vi "FPGAsimpleTDC.vi"() -> ()   [LabVIEW 2017]
uses:
  <vilib>/Platform/TimedLoop/XDataNode/timing_clust.ctl
  <vilib>/Platform/TimedLoop/XDataNode/nitl_modes.ctl
  <vilib>/Platform/TimedLoop/XDataNode/wakeup.ctl
  <vilib>/rvi/Emulation/niFpgaGetClockAttributes.vi
  <vilib>/rvi/Emulation/niFpgaSctlEmulationGetInTimedLoop.vi
  <vilib>/rvi/Emulation/niFpgaEmulationReportErrorSimple.vi
  <vilib>/rvi/Emulation/niFpgaProcessEmulError.vi
  <vilib>/rvi/Emulation/niFpgaCriticalErrorInLSC.vi
  <vilib>/rvi/eio/common/nirviEmuTemplateMethod_errors.vi
  <vilib>/rvi/DataTransferAndStorage/Container/Common/niFpgaContainerExecOnDevCompGetState.vi
  <vilib>/rvi/Emulation/niFpgaEmulationIsFPGAContextNoSignature.vi
  <vilib>/rvi/errors/niFpgaSetErrorForExecOnDevCompSimple.vi
  <vilib>/rvi/eio/common/nirviEmuReportErrorAndStop.vi
  <vilib>/rvi/DataTransferAndStorage/Container/Common/niFpgaContainerGetUniqueNameForEmu.vi
  <vilib>/rvi/FIFO/Fifo_Resource/nirvififoEmulationSetSize.vi
  <vilib>/rvi/FIFO/Fifo_Resource/nirviFifoEmulationQueueMgr.vi
  <instcachedir>/0/nirviFifoEmulationQueueMgr_E5CAEC123FF24DC58D834DCA3CDAA9B5.lvgen/nirviFifoEmulationQueueMgr_E5CAEC123FF24DC58D834DCA3CDAA9B5_001.vi
  <vilib>/rvi/FIFO/Fifo_Resource/nirvififoEmulationDetermineInputValidOut.vi
  <vilib>/rvi/FIFO/Fifo_Resource/nirvififoEmulationCreateLock.vi
  <vilib>/rvi/FIFO/Fifo_Resource/nirvififoEmulationObtainLock.vi
  <vilib>/rvi/FIFO/Fifo_Resource/nirvififoEmulationReleaseLock.vi
  <vilib>/rvi/occurrence/nirviWaitOnOccurrenceBase.vi
  <vilib>/rvi/errors/nirviReportUnexpectedCaseInternalError.vi
  <vilib>/rvi/errors/nirviReportUnexpectedCaseInternalError (U32).vi
  <vilib>/Utility/error.llb/Clear Errors.vi
  <vilib>/rvi/interface/RandomDataEmulation/niFpgaRandomDataHandleErrors.vi
  <vilib>/Platform/TimedLoop/XDataNode/XDataNode.xnode
  <vilib>/eio/EIONode/EIONode.xnode
  <vilib>/rvi/DataTransferAndStorage/Container/XNode/niFpgaContainer.xnode
  <vilib>/rvi/FIFO/Fifo_Resource/niFpgaFifoEmulationRefIn.vi
  <vilib>/Platform/TimedLoop/XDataNode/XDNodeRunTimeDep.lvlib
panel:
  in  "Acquire times":bool
  in  "N photons":u32
  out "new data":bool=TRUE
  out "tau":u32
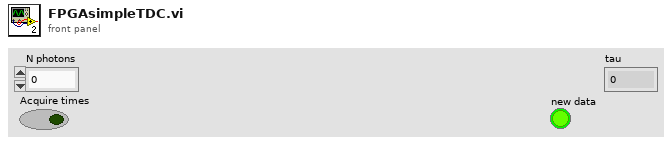
[diagram p1: front panel]
types:
  T1 = typedef "XDNodeRunTimeDep.lvlib/timing_clust.ctl" = cluster{"Expected End [f-1]":u64, "Actual End [f-1]":u64, "Finished Late? [f-1]":bool, "Expected End [i-1]":u64, "Actual End [i-1]":u64, "Finished Late? [i-1]":bool, "Expected Start [i]":u64, "Actual Start [i]":u64, "Expected Start [f]":u64, "Actual Start [f]":u64, "Source Name":string, "Structure Name":string, "Period":i64, "Deadline":i64, "Offset":i64, "Start":i64, "Priority":i32, "Timeout":i32, "Mode":T2, "Wakeup Reason":T3, "Error":errorcluster, "Source Type":string, "Secondary Source Type":string, "Global End Time":u64, "Global Start Time":u64, "Frame Duration":u64, "Iteration Duration":u64, "Assigned CPU":i32, "I/O Scan Engine Mode":u32}
  T2 = typedef "XDNodeRunTimeDep.lvlib/nitl_modes.ctl" = enum32{"No Change", "Process missed periods, maintain original phase", "Discard missed periods, maintain original phase", "Process missed periods, ignore original phase", "Discard missed periods, ignore original phase"}
  T3 = typedef "XDNodeRunTimeDep.lvlib/wakeup.ctl" = enum32{"Normal", "Aborted", "Asynchronous wakeup", "Timing source error", "Timed loop error", "Timeout"}
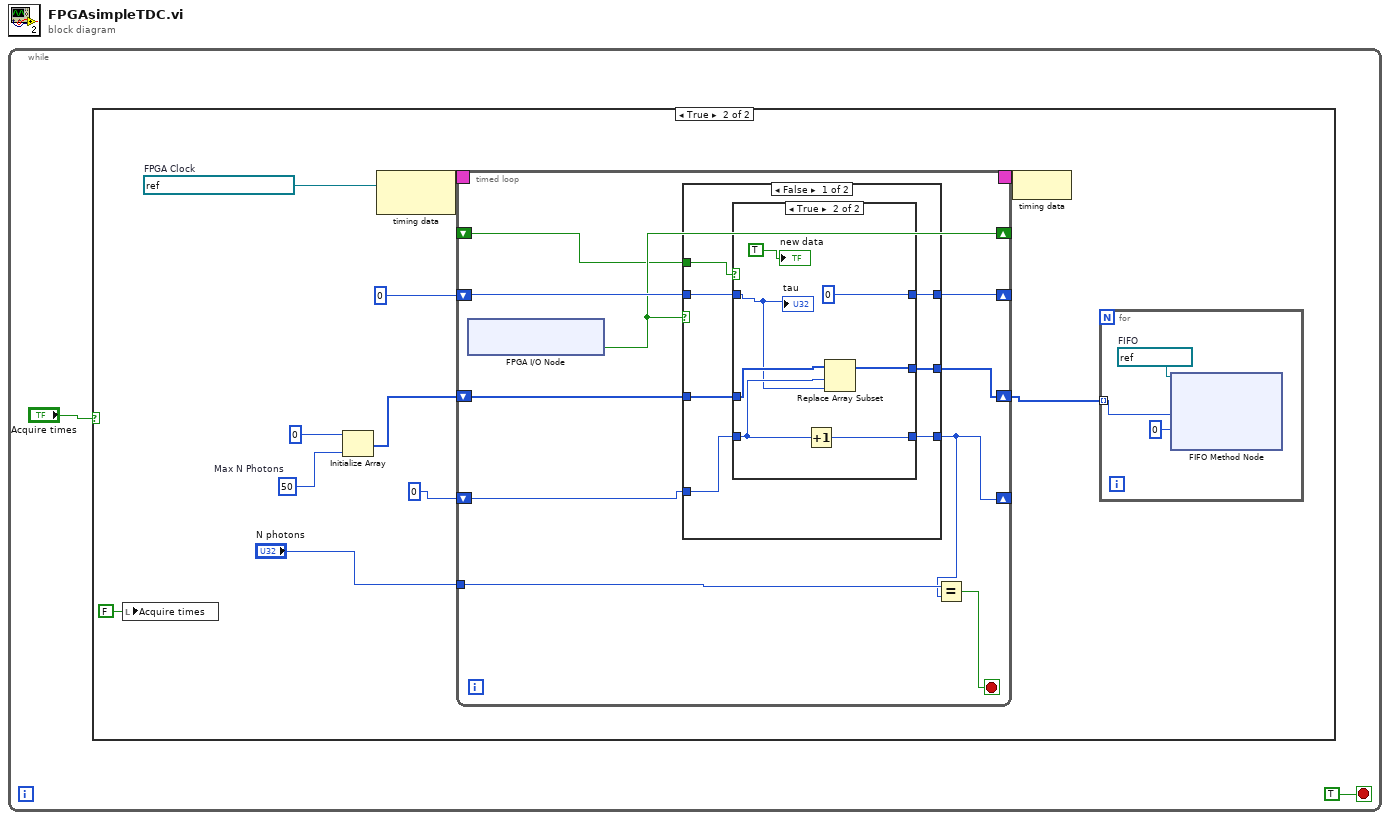
[diagram p0: block diagram]
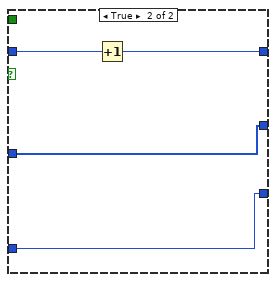
[diagram p4: hidden frame]
diagram:
  n1 = while {
    stop <- TRUE stop-if-true
    n2 = case shown="True" "Acquire times" {
      frame False {
      }
      frame True {
        w3 = u32 50  # Max N Photons
        w10 = refnum<k21> "40 MHz Onboard Clock"  # FPGA Clock
        n3 = local write "Acquire times"(FALSE ("Acquire times")) -> ()
        n4 = Initialize Array(u32 0, w3) -> (w6:u32[])
        n5 = node-c288(w10) -> (w13:T1)
        n6 = timed-loop {
          timing: w13 -> [_]
          timing-out: [_] -> w12
          shift-right: [w25] -> _
          shift-left: u32 0 -> [w26]
          shift-right: [w24] -> _
          shift-left: _ -> [w23]
          shift-right: [w22] -> w11
          shift-left: w6 -> [w21]
          tunnel: "N photons" -> [w19]
          shift-right: [w17] -> _
          shift-left: u32 0 -> [w18]
          stop <- w20 stop-if-true
          n7 = xnode "FPGA I/O Node"() -> ("Connector0/DIO5"=w24:bool)  [unwired: 1 in, 1 out]
          n8 = case shown="False" w24 {
            tunnel: w26 -> [w32 w47]
            tunnel: [w31 w46] -> w25
            tunnel: w23 -> [w33 _]
            tunnel: w21 -> [w30 w45]
            tunnel: [w29 w45] -> w22
            tunnel: w18 -> [w28 w44]
            tunnel: [w27 w44] -> w17
            frame False {
              n9 = case shown="True" w33 {
                tunnel: w32 -> [w36 w38]
                tunnel: [w36 i16 0] -> w31
                tunnel: w30 -> [w35 w40]
                tunnel: [w35 w37] -> w29
                tunnel: w28 -> [w34 w39]
                tunnel: [w34 w41] -> w27
                frame False {
                }
                frame True {
                  n10 = Increment(x=w39) -> (x+1=w41:u32)
                  n11 = Replace Array Subset(array=w40, new element=w38, index=w39) -> (w37:u32[])
                  "new data" <- TRUE ("new data")
                  "tau" <- w38
                }
              }
            }
            frame True {
              n12 = Increment(x=w47) -> (x+1=w46:u32)
            }
          }
          n13 = Equal?(x=w19, y=w17) -> (x = y?=w20:bool)
        }
        n14 = node-c288(w12) -> ()
        n15 = for {
          tunnel: w11 -> [w15] mode=indexing
          w16 = refnum<k21> "U32 FIFO"  # FIFO
          n16 = xnode ("FIFO Method Node")("Element"=w15, "Timeout"=0, "FIFO In"=w16) -> ()  [unwired: 2 out]
        }
      }
    }
  }
